vi "set_zero.vi"(8 "error in (no error)":errorcluster, 11 "BMC in":refnum<class "BMC.lvclass">) -> (0 "error out":errorcluster, 3 "BMC out":refnum<class "BMC.lvclass">)   [LabVIEW 2012, in "BMC.lvclass"]
uses:
  BMC.lvclass
  BMC.lvclass/BMC.ctl
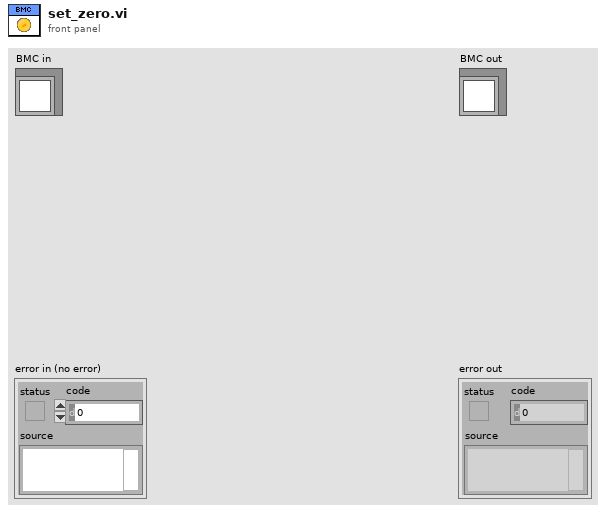
[diagram p1: front panel]
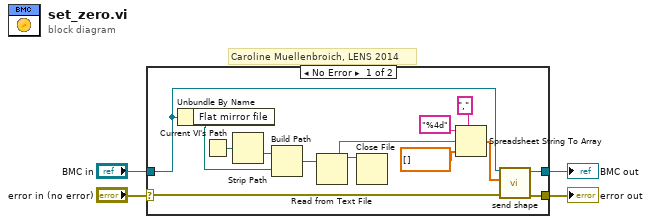
[diagram p0: block diagram]
diagram:
  # "Caroline Muellenbroich, LENS 2014"
  n1 = case shown="No Error" "error in (no error)" {
    selector: "error in (no error)" -> [w8 w20]
    tunnel: [w6 w20] -> w3
    tunnel: [w5 w19] -> w1
    tunnel: "BMC in" -> [w7 w19]
    frame No Error {
      n2 = Unbundle By Name(w7) -> ("Flat mirror file"=w10:path)
      n3 = Current VI's Path() -> (path=w15:path)
      n4 = Strip Path(path=w15) -> (stripped path=w16:path)  [unwired: 1 out]
      n5 = Build Path(base path=w16, name or relative path=w10) -> (appended path=w14:path)
      n6 = Read from Text File(file (use dialog)=w14) -> (refnum out=w17:refnum<file>, text=w18:string)  [unwired: 1 in, 4 out]
      n7 = Close File(refnum=w17) -> ()  [unwired: 1 in, 2 out]
      n8 = Spreadsheet String To Array(delimiter (Tab)=",", format string="%4d", spreadsheet string=w18, array type (2D Dbl)=dbl[] [] ("run time Cluster.1x160  Voltage Map")) -> (array=w9:dbl[])
      n9 = call-dynamic "send shape.vi"("error in (no error)"=w8, "1x160 Voltage Map"=w9, "BMC in"=w7) -> ("error out"=w6:errorcluster, "BMC out"=w5:refnum<class "BMC.lvclass">)  [unwired: 7 in]
    }
    frame Error {
    }
  }
  "error out" <- w3
  "BMC out" <- w1
